vi "Serial send & receive.vi"(9 "Command":string, 10 "delay before read (ms)":u32, 11 "VISA Refnum in":refnum<visa-resource-name>) -> (2 "read buffer":string, 3 "Bytes at Port":u32)   [LabVIEW 2016]
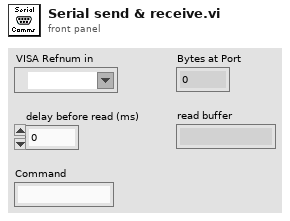
[diagram p1: front panel]
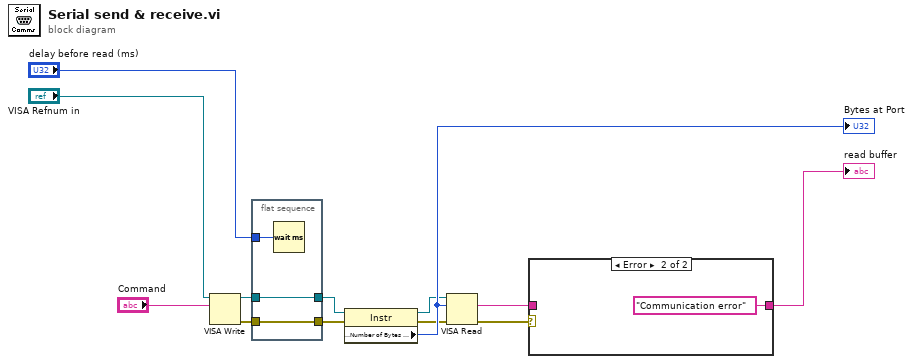
[diagram p0: block diagram]
diagram:
  n1 = VISA Write(VISA resource name="VISA Refnum in", write buffer="Command") -> (VISA resource name out=w8:refnum<visa-resource-name>, error out=w10:errorcluster)  [unwired: 1 in, 1 out]
  n2 = flat-sequence {
    tunnel: w10 -> [w16]
    tunnel: [w16] -> w9
    tunnel: w8 -> [w15]
    tunnel: [w15] -> w7
    tunnel: "delay before read (ms)" -> [w14]
    frame #0 {
      n3 = Wait (ms)(milliseconds to wait=w14) -> ()  [unwired: 1 out]
    }
  }
  n4 = property class="Instr"(reference=w7, error in=w9) -> (reference out=w5:refnum<visa-resource-name>, error out=w4:errorcluster, "Serial Settings:Number of Bytes at Serial Port"=w11:u32)
  "Bytes at Port" <- w11
  n5 = VISA Read(VISA resource name=w5, byte count=w11, error in (no error)=w4) -> (read buffer=w2:string, error out=w3:errorcluster)  [unwired: 2 out]
  n6 = case shown="Error" w3 {
    tunnel: w2 -> [w17 _]
    tunnel: [w17 "Communication error" ("read buffer")] -> w1
    frame No Error {
    }
    frame Error {
    }
  }
  "read buffer" <- w1
